vi "Interpolate Points (Number).vi"(1 "End Point":cluster{"X":dbl, "Y":dbl}, 2 "Number of Points":dbl, 3 "Start Point":cluster{"X":dbl, "Y":dbl}) -> (0 "Output Point Array":cluster{"X":dbl, "Y":dbl}[](array[cluster]))   [LabVIEW 2019]
doc: "This VI interpolates at specified intervals between two points."
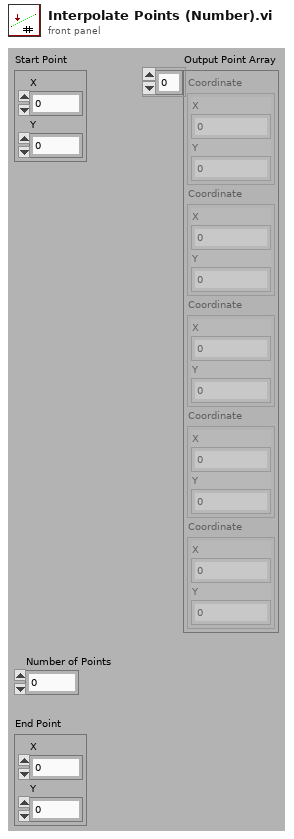
[diagram p1: front panel]
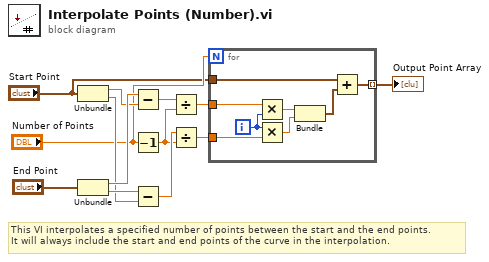
[diagram p0: block diagram]
diagram:
  # "This VI interpolates a specified number of points between the start and the end points.\nIt will always include the start and end points of the curve in the interpolation."
  n1 = Unbundle("Start Point") -> ("X"=w6:dbl, "Y"=w5:dbl)
  n2 = Unbundle("End Point") -> ("X"=w8:dbl, "Y"=w7:dbl)
  n3 = Subtract(x=w8, y=w6) -> (x-y=w13:dbl)
  n4 = Decrement(x="Number of Points") -> (x-1=w9:dbl)
  n5 = Subtract(x=w7, y=w5) -> (x-y=w12:dbl)
  n6 = Divide(x=w13, y=w9) -> (x/y=w11:dbl)
  n7 = Divide(x=w12, y=w9) -> (x/y=w10:dbl)
  n8 = for {
    N: "Number of Points" -> [_]
    tunnel: w11 -> [w21]
    tunnel: w10 -> [w19]
    tunnel: "Start Point" -> [w15]
    tunnel: [w14] -> w1 mode=indexing
    i -> [w20]
    n9 = Multiply(x=w21, y=w20) -> (x*y=w18:dbl)
    n10 = Multiply(x=w20, y=w19) -> (x*y=w17:dbl)
    n11 = Bundle(w18, w17) -> (w16:cluster{dbl, dbl})  [unwired: 1 in]
    n12 = Add(x=w15, y=w16) -> (x+y=w14:cluster{dbl, dbl})
  }
  "Output Point Array" <- w1
